vi "hydrolyse_reactor_run.vi"(11 "#":i32) -> ()   [LabVIEW 2019]
uses:
  <vilib>/Utility/sysdir.llb/System Directory Type.ctl
  lib/libSimulationControl/libSimulationControl.lvlib
panel:
  out "path":path
  out "spec":string
  out "current_time":dbl
  # "*******************************************************************\nBiogas Plant Control\n\nAuthor: Paul Zügel\nGCSC-Frankfurt am Main 2020\n\n*******************************************************************"
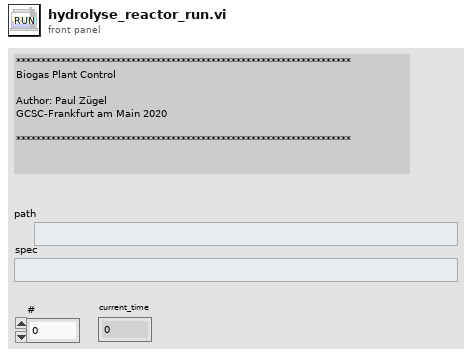
[diagram p1: front panel]
types:
  T1 = typedef "System Directory Type.ctl" = i32
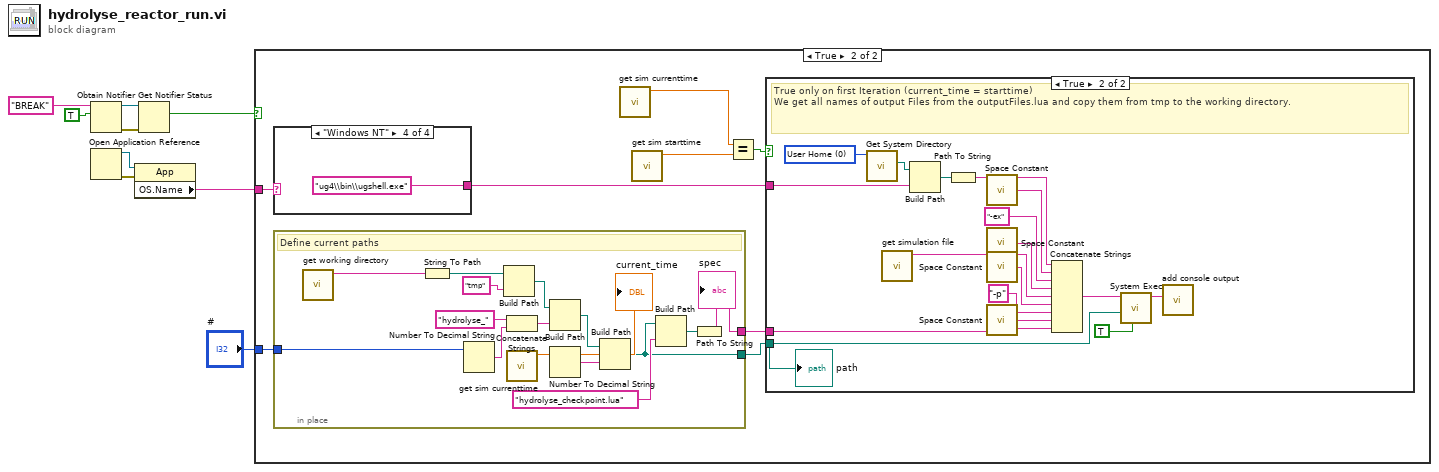
[diagram p0: block diagram]
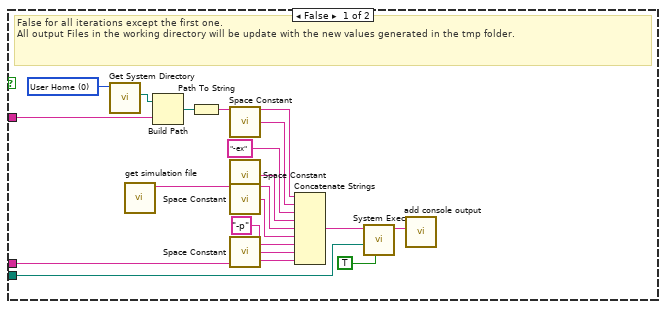
[diagram p3: hidden frame]
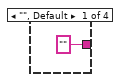
[diagram p4: hidden frame]
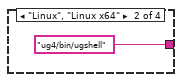
[diagram p5: hidden frame]
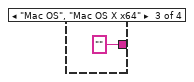
[diagram p6: hidden frame]
diagram:
  n1 = Obtain Notifier(name (unnamed)="BREAK", notification data type=TRUE) -> (notifier out=w7:refnum<notifier>, error out=w6:errorcluster)  [unwired: 2 in, 1 out]
  n2 = Open Application Reference() -> (0:w3:errorcluster, 3:w4:refnum<vi>)  [unwired: 4 in]
  n3 = property class="App"(reference=w4, error in=w3) -> ("OS.Name"=w2:string)  [unwired: 2 out]
  n4 = Get Notifier Status(notifier=w7, error in (no error)=w6) -> (current notification=w5:bool)  [unwired: 4 out]
  n5 = case shown="True" w5 {
    tunnel: w2 -> [_ w17]
    tunnel: "#" -> [_ w12]
    frame False {
    }
    frame True {
      n6 = case shown="\"Windows NT\"" w17 {
        tunnel: ["" ("return type") "ug4/bin/ugshell" ("name or relative path") "" ("return type") "ug4\\bin\\ugshell.exe" ("name or relative path")] -> w13
        frame "", Default {
        }
        frame "Linux", "Linux x64" {
        }
        frame "Mac OS", "Mac OS X x64" {
        }
        frame "Windows NT" {
        }
      }
      n7 = in-place {
        in-place-border: w12 -> [w27]
        in-place-border: [w19] -> w11
        in-place-border: [w18] -> w10
        # "Define current paths"
        n8 = call "get working directory.vi"() -> ("function return"=w32:string)  [unwired: 10 in, 1 out]
        n9 = String To Path(string=w32) -> (path=w31:path)
        n10 = Number To Decimal String(number=w27) -> (decimal integer string=w26:string)  [unwired: 1 in]
        n11 = Build Path(base path=w31, name or relative path="tmp") -> (appended path=w29:path)
        n12 = Concatenate Strings("hydrolyse_" ("string"), w26) -> (w25:string)
        n13 = call "get sim currenttime.vi"() -> ("current_time"=w21:dbl)  [unwired: 10 in, 1 out]
        "current_time" <- w21
        n14 = Build Path(base path=w29, name or relative path=w25) -> (appended path=w22:path)
        n15 = Number To Decimal String(number=w21) -> (decimal integer string=w20:string)  [unwired: 1 in]
        n16 = Build Path(base path=w22, name or relative path=w20) -> (appended path=w19:path)
        n17 = Build Path(base path=w19, name or relative path="hydrolyse_checkpoint.lua") -> (appended path=w23:path)
        n18 = Path To String(path=w23) -> (string=w18:string)
        "spec" <- w18
      }
      n19 = call "get sim currenttime.vi"() -> ("current_time"=w16:dbl)  [unwired: 10 in, 1 out]
      n20 = call "get sim starttime.vi"() -> ("sim_starttime"=w15:dbl)  [unwired: 10 in, 1 out]
      n21 = Equal?(x=w16, y=w15) -> (x = y?=w14:bool)
      n22 = case shown="True" w14 {
        tunnel: w13 -> [w35 w65]
        tunnel: w11 -> [w34 w51]
        tunnel: w10 -> [w33 w50]
        frame False {
          w41 = T1 0 items=["User Home"=0, "User Desktop"=1, "User Documents"=2, "User Application Data"=3, "User Preferences"=4, "User Temporary"=5, "Public Documents"=6, "Public Application Data"=7, "Public Preferences"=8, "Public Cache"=13, "System Core Libraries"=9, "System Installed Libraries"=10, "Application Files"=11, "Boot Volume Root"=12] ("system directory type")
          # "False for all iterations except the first one.\nAll output Files in the working directory will be update with the new values generated in the tmp folder."
          n23 = call <vilib>:"Get System Directory.vi"("system directory type"=w41) -> ("system directory"=w48:path)  [unwired: 10 in]
          n24 = call "get simulation file.vi"() -> ("function return"=w38:string)  [unwired: 10 in, 1 out]
          n25 = Build Path(base path=w48, name or relative path=w35) -> (appended path=w46:path)
          n26 = Path To String(path=w46) -> (string=w42:string)
          n27 = call <vilib>:"Space Constant.vi"() -> ("String"=w43:string)
          n28 = call <vilib>:"Space Constant.vi"() -> ("String"=w44:string)
          n29 = call <vilib>:"Space Constant.vi"() -> ("String"=w45:string)
          n30 = call <vilib>:"Space Constant.vi"() -> ("String"=w49:string)
          n31 = Concatenate Strings(w42, w43, "-ex" ("command line"), w44, w38, w45, "-p" ("command line"), w49, w33) -> (w47:string)
          n32 = call <vilib>:"System Exec.vi"("run minimized? (F)"=TRUE, "working directory"=w34, "command line"=w47) -> ("standard output"=w36:string)  [unwired: 5 in, 3 out]
          n33 = call "add console output.vi"("add_to_console"=w36) -> ()  [unwired: 11 in]
        }
        frame True {
          w56 = T1 0 items=["User Home"=0, "User Desktop"=1, "User Documents"=2, "User Application Data"=3, "User Preferences"=4, "User Temporary"=5, "Public Documents"=6, "Public Application Data"=7, "Public Preferences"=8, "Public Cache"=13, "System Core Libraries"=9, "System Installed Libraries"=10, "Application Files"=11, "Boot Volume Root"=12] ("system directory type")
          # "True only on first Iteration (current_time = starttime)\nWe get all names of output Files from the outputFiles.lua and copy them from tmp to the working directory."
          n34 = call <vilib>:"Get System Directory.vi"("system directory type"=w56) -> ("system directory"=w63:path)  [unwired: 10 in]
          n35 = call "get simulation file.vi"() -> ("function return"=w53:string)  [unwired: 10 in, 1 out]
          n36 = Build Path(base path=w63, name or relative path=w65) -> (appended path=w61:path)
          n37 = Path To String(path=w61) -> (string=w57:string)
          n38 = call <vilib>:"Space Constant.vi"() -> ("String"=w58:string)
          n39 = call <vilib>:"Space Constant.vi"() -> ("String"=w59:string)
          n40 = call <vilib>:"Space Constant.vi"() -> ("String"=w60:string)
          n41 = call <vilib>:"Space Constant.vi"() -> ("String"=w64:string)
          n42 = Concatenate Strings(w57, w58, "-ex" ("command line"), w59, w53, w60, "-p" ("command line"), w64, w50) -> (w62:string)
          n43 = call <vilib>:"System Exec.vi"("run minimized? (F)"=TRUE, "working directory"=w51, "command line"=w62) -> ("standard output"=w66:string)  [unwired: 5 in, 3 out]
          n44 = call "add console output.vi"("add_to_console"=w66) -> ()  [unwired: 11 in]
          "path" <- w51
        }
      }
    }
  }
